vi "Fetch (NT Scalar).vi"(7 "PV name":string, 8 "error in":errorcluster, 10 "default value":refnum<class "NT Scalar.lvclass">, 11 "Server in":refnum<class "Server.lvclass">) -> (0 "error out":errorcluster, 2 "value":refnum<class "NT Scalar.lvclass">, 3 "Server out":refnum<class "Server.lvclass">)   [LabVIEW 2020, in "PV Access.lvlib" / "PVA Server.lvlib" / "Server.lvclass"]
uses:
  Server.lvclass
  PV Data/NT Scalar/NT Scalar.lvclass
  PV Data/PV Data/PV Data.lvclass
  Source/Source.lvclass
  Server.lvclass/Server.ctl
  C:/Users/eyw68381/source/repos/pvaccess-labview/labview/source/PV Data/NT Base/NT Base.lvclass
  C:/Users/eyw68381/source/repos/pvaccess-labview/labview/source/PV Data/NT Scalar/NT Scalar.lvclass
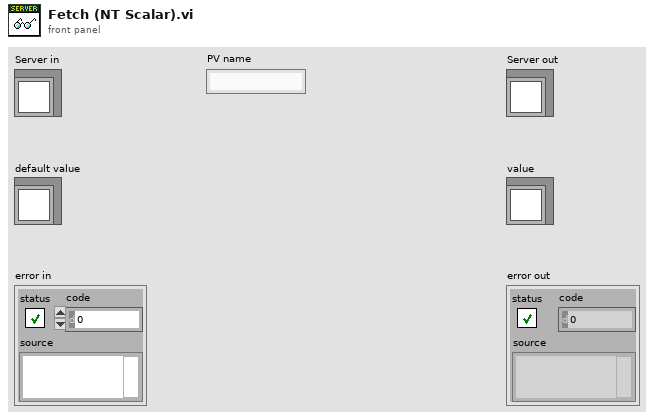
[diagram p1: front panel]
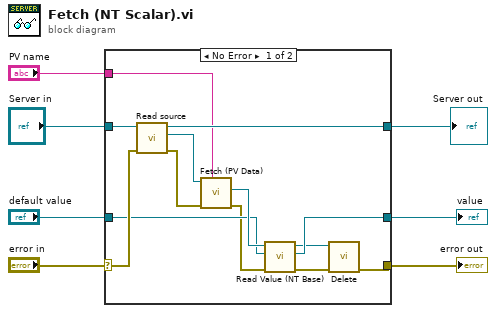
[diagram p0: block diagram]
diagram:
  n1 = case shown="No Error" "error in" {
    selector: "error in" -> [w20 w21]
    tunnel: [w11 w21] -> w7
    tunnel: "PV name" -> [w17 _]
    tunnel: "Server in" -> [w19 w23]
    tunnel: [w18 w23] -> w3
    tunnel: "default value" -> [w13 w22]
    tunnel: [w12 w22] -> w1
    frame No Error {
      n2 = call "Read source.vi"("error in (no error)"=w20, "Server in"=w19) -> ("error out"=w16:errorcluster, "Source"=w15:refnum<class "Source.lvclass">, "Server out"=w18:refnum<class "Server.lvclass">)  [unwired: 7 in]
      n3 = call "Fetch (PV Data).vi"("PV name"=w17, "error in"=w16, "Source in"=w15) -> ("error out"=w8:errorcluster, "PV Data out"=w14:refnum<class "PV Data.lvclass">)  [unwired: 6 in, 1 out]
      n4 = call "Read Value (NT Base).vi"("error in (no error)"=w8, "default value"=w13, "PV Data in"=w14) -> ("error out"=w10:errorcluster, "value"=w12:refnum<class "NT Scalar.lvclass">, "PV Data out"=w9:refnum<class "PV Data.lvclass">)  [unwired: 6 in]
      n5 = call "Delete.vi"("error in (no error)"=w10, "PV Data in"=w9) -> ("error out"=w11:errorcluster)  [unwired: 9 in]
    }
    frame Error {
    }
  }
  "Server out" <- w3
  "error out" <- w7
  "value" <- w1
